vi "IE Save dialog build path.vi"(6 "New String":string, 8 "error in (no error)":errorcluster, 10 "Start tag":string, 11 "Tree Refnum":refnum<vi>) -> (0 "error out":errorcluster, 3 "New path":path)   [LabVIEW 2020]
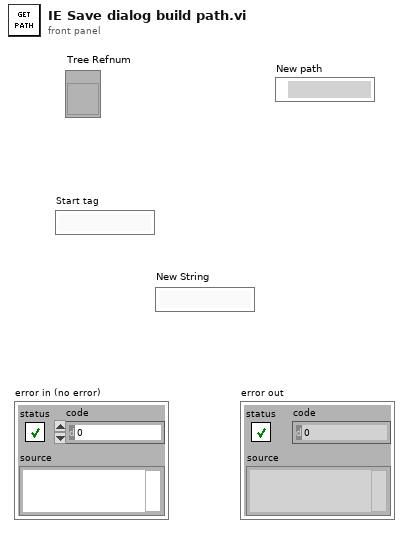
[diagram p1: front panel]
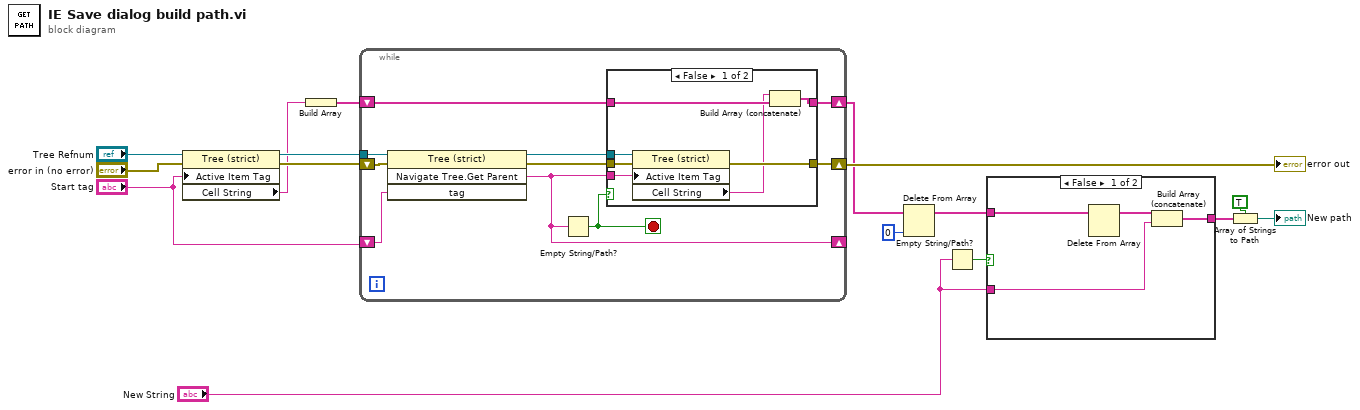
[diagram p0: block diagram]
diagram:
  n1 = property class="Tree (strict)"(reference="Tree Refnum", error in="error in (no error)", "Active Item Tag"="Start tag") -> (reference out=w11:refnum<vi>, error out=w10:errorcluster, "Cell String"=w9:string)
  n2 = Build Array(w9) -> (w8:string[])
  n3 = while {
    tunnel: w11 -> [w26]
    shift-right: [w22] -> _
    shift-left: "Start tag" -> [w25]
    shift-right: [w20] -> w14
    shift-left: w10 -> [w21]
    shift-right: [w17] -> w7
    shift-left: w8 -> [w18]
    stop <- w19 stop-if-true
    n4 = invoke class="Tree (strict)" method="Navigate Tree.Get Parent"(reference=w26, error in=w21, "tag"=w25) -> (reference out=w24:refnum<vi>, error out=w23:errorcluster, "Navigate Tree:Get Parent"=w22:string)  [unwired: 1 in, 1 out]
    n5 = Empty String/Path?(string/path=w22) -> (empty?=w19:bool)
    n6 = case shown="False" w19 {
      tunnel: w24 -> [w33 _]
      tunnel: w23 -> [w32 w35]
      tunnel: w22 -> [w31 _]
      tunnel: [w30 w35] -> w20
      tunnel: w18 -> [w29 w34]
      tunnel: [w27 w34] -> w17
      frame False {
        n7 = property class="Tree (strict)"(reference=w33, error in=w32, "Active Item Tag"=w31) -> (error out=w30:errorcluster, "Cell String"=w28:string)  [unwired: 1 out]
        n8 = Build Array (concatenate)(w28, w29) -> (w27:string[])
      }
      frame True {
      }
    }
  }
  "error out" <- w14
  n9 = Delete From Array(array=w7, index=0) -> (array with subset deleted=w5:string[])  [unwired: 1 in, 1 out]
  n10 = Empty String/Path?(string/path="New String") -> (empty?=w12:bool)
  n11 = case shown="False" w12 {
    tunnel: [w39 w40] -> w6
    tunnel: "New String" -> [w37 _]
    tunnel: w5 -> [w38 w40]
    frame False {
      n12 = Delete From Array(array=w38) -> (array with subset deleted=w36:string[])  [unwired: 2 in, 1 out]
      n13 = Build Array (concatenate)(w36, w37) -> (w39:string[])
    }
    frame True {
    }
  }
  n14 = Array of Strings to Path(0:w6, 1:TRUE ("relative")) -> (2:→"New path":path)
